vi "SetRunSeq_popup.vi"(8 "error in (no error)":errorcluster, 9 "Input Line Command":string, 10 "platform":u16(ring) items=["Mac", "PC"]) -> (0 "error out":errorcluster, 1 "Output Line Command":string, 2 "Cancel":bool)   [LabVIEW 2019]
panel:
  in  "Cancel button":bool
  in  "OK Button":bool
  in  "Path":path
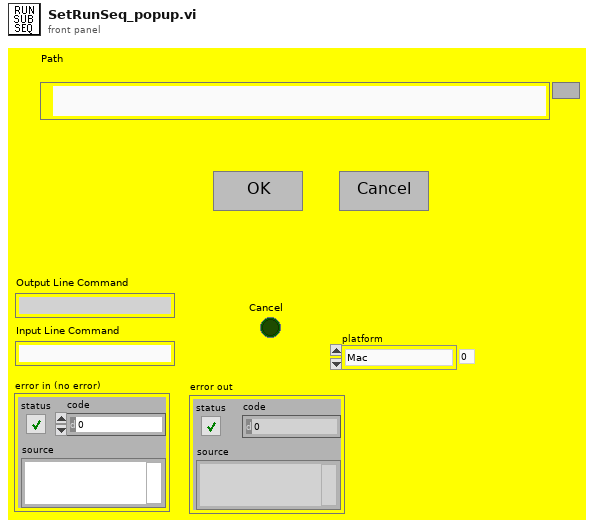
[diagram p1: front panel]
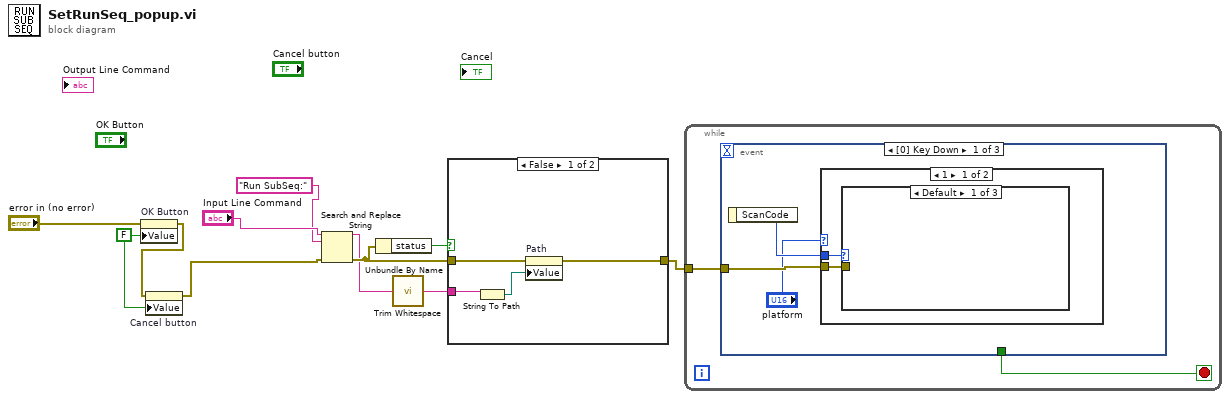
[diagram p0: block diagram]
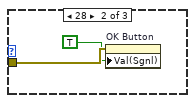
[diagram p2: hidden frame]
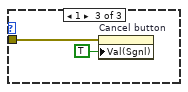
[diagram p3: hidden frame]
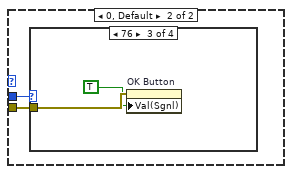
[diagram p4: hidden frame]
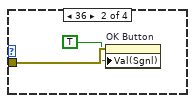
[diagram p6: hidden frame]
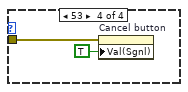
[diagram p7: hidden frame]
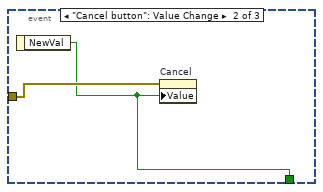
[diagram p8: hidden frame]
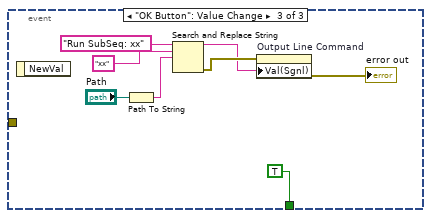
[diagram p9: hidden frame]
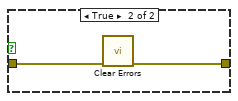
[diagram p10: hidden frame]
diagram:
  w9 = FALSE ("OK Button")
  n1 = property on="OK Button" class="Bool (strict)"(error in="error in (no error)", "Value"=w9) -> (error out=w10:errorcluster)  [unwired: 1 in, 1 out]
  n2 = property on="Cancel button" class="Bool (strict)"(error in=w10, "Value"=w9) -> (error out=w4:errorcluster)  [unwired: 1 in, 1 out]
  n3 = Search and Replace String(input string="Input Line Command", search string="Run SubSeq:" ("format string"), error in=w4) -> (result string=w2:string, error out=w3:errorcluster)  [unwired: 5 in, 2 out]
  n4 = Unbundle By Name(w3) -> ("status"=w8:bool)
  n5 = call <vilib>:"Trim Whitespace.vi"("string"=w2) -> ("trimmed string"=w1:string)  [unwired: 1 in]
  n6 = case shown="False" w8 {
    tunnel: w3 -> [w15 w17]
    tunnel: [w14 w16] -> w7
    tunnel: w1 -> [w13 _]
    frame False {
      n7 = String To Path(string=w13) -> (path=w12:path)
      n8 = property on="Path" class="Path"(error in=w15, "Value"=w12) -> (error out=w14:errorcluster)  [unwired: 1 in, 1 out]
    }
    frame True {
      n9 = call <vilib>:"Clear Errors.vi"("error in (no error)"=w17) -> ("error out"=w16:errorcluster)  [unwired: 5 in, 1 out]
    }
  }
  n10 = while {
    tunnel: w7 -> [w19]
    stop <- w18 stop-if-true
    n11 = event shown="[0] Key Down" {
      selector: _ -> [_ _ _]
      dyn-events: _ -> [_ _ _]
      timeout: _ -> [_ _ _]
      tunnel: w19 -> [w21 w38 _]
      tunnel: [_ w37 TRUE] -> w18
      event Key Down {
        n12 = event-data() -> ("ScanCode"=w22:i16)  [unwired: 1 in]
        n13 = case shown="1" "platform" {
          tunnel: w22 -> [w24 w30]
          tunnel: w21 -> [w23 w29]
          frame 1 {
            n14 = case shown="Default" w24 {
              tunnel: w23 -> [_ w26 w28]
              frame Default {
              }
              frame 28 {
                n15 = property on="OK Button" class="Bool (strict)"(error in=w26, "Val(Sgnl)"=TRUE ("Value (Signaling)")) -> ()  [unwired: 1 in, 2 out]
              }
              frame 1 {
                n16 = property on="Cancel button" class="Bool (strict)"(error in=w28, "Val(Sgnl)"=TRUE ("Value (Signaling)")) -> ()  [unwired: 1 in, 2 out]
              }
            }
          }
          frame 0, Default {
            n17 = case shown="76" w30 {
              tunnel: w29 -> [_ w32 w34 w36]
              frame Default {
              }
              frame 36 {
                n18 = property on="OK Button" class="Bool (strict)"(error in=w32, "Val(Sgnl)"=TRUE ("Value (Signaling)")) -> ()  [unwired: 1 in, 2 out]
              }
              frame 76 {
                n19 = property on="OK Button" class="Bool (strict)"(error in=w34, "Val(Sgnl)"=TRUE ("Value (Signaling)")) -> ()  [unwired: 1 in, 2 out]
              }
              frame 53 {
                n20 = property on="Cancel button" class="Bool (strict)"(error in=w36, "Val(Sgnl)"=TRUE ("Value (Signaling)")) -> ()  [unwired: 1 in, 2 out]
              }
            }
          }
        }
      }
      event "Cancel button": Value Change {
        n21 = event-data() -> ("NewVal"=w37:bool)  [unwired: 1 in]
        n22 = property on="Cancel" class="Bool (strict)"(error in=w38, "Value"=w37) -> ()  [unwired: 1 in, 2 out]
      }
      event "OK Button": Value Change {
        n23 = event-data() -> ()  [unwired: 1 in, 1 out]
        n24 = Path To String(path="Path") -> (string=w39:string)
        n25 = Search and Replace String(input string="Run SubSeq: xx", search string="xx", replace string=w39) -> (result string=w42:string, error out=w43:errorcluster)  [unwired: 5 in, 2 out]
        n26 = property on="Output Line Command" class="Str"(error in=w43, "Val(Sgnl)"=w42) -> (error out=→"error out":errorcluster)  [unwired: 1 in, 1 out]
      }
    }
  }
